vi "save_config_file.vi"(8 "error in (no error)":errorcluster, 9 "config cluster variant":variant, 11 "StageMG100204SutterMP285 in":refnum<class "StageMG100204SutterMP285.lvclass">=refnum) -> (0 "error out":errorcluster, 3 "StageMG100204SutterMP285 out":refnum<class "StageMG100204SutterMP285.lvclass">)   [LabVIEW 2010, in "StageMG100204SutterMP285.lvclass"]
uses:
  StageMG100204SutterMP285.lvclass
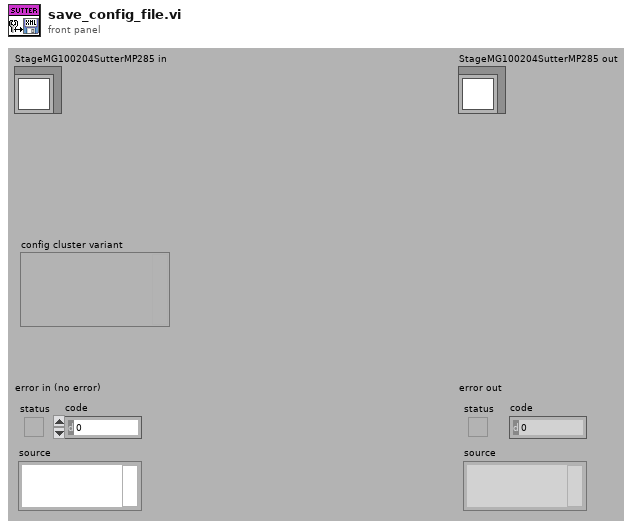
[diagram p1: front panel]
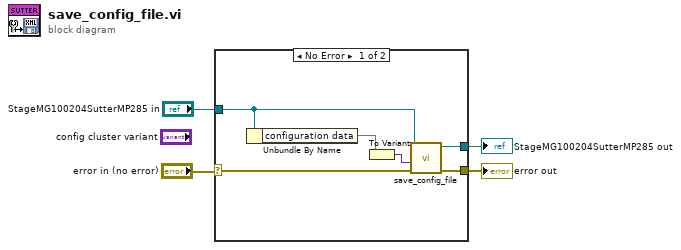
[diagram p0: block diagram]
diagram:
  n1 = case shown="No Error" "error in (no error)" {
    selector: "error in (no error)" -> [w5 w11]
    tunnel: [w10 w11] -> w3
    tunnel: "StageMG100204SutterMP285 in" -> [w8 w12]
    tunnel: [w9 w12] -> w1
    frame No Error {
      n2 = Unbundle By Name(w8) -> ("configuration data"=w6)
      n3 = To Variant(anything=w6) -> (Variant=w7:variant)
      n4 = call-parent "save_config_file.vi"("error in (no error)"=w5, "config cluster variant"=w7, "GenericPlugin in"=w8) -> ("error out"=w10:errorcluster, "GenericPlugin out"=w9:refnum<class "StageMG100204SutterMP285.lvclass">)  [unwired: 7 out]
    }
    frame Error {
    }
  }
  "error out" <- w3
  "StageMG100204SutterMP285 out" <- w1
